vi "In Place Write String.vi"(8 "error in (no error)":errorcluster, 9 "offset (0)":i64, 10 "string in":string, 11 "pointer in":u64) -> (0 "error out":errorcluster, 1 "offset out":i64, 2 "string out":string, 3 "pointer out":u64)   [LabVIEW 2013, in "Linux RT IPC.Shared Memory.lvlib"]
uses:
  Linux RT IPC.Shared Memory.lvlib
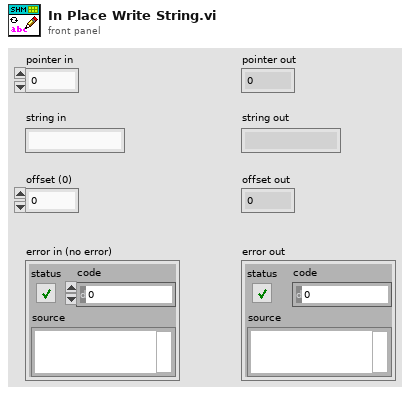
[diagram p1: front panel]
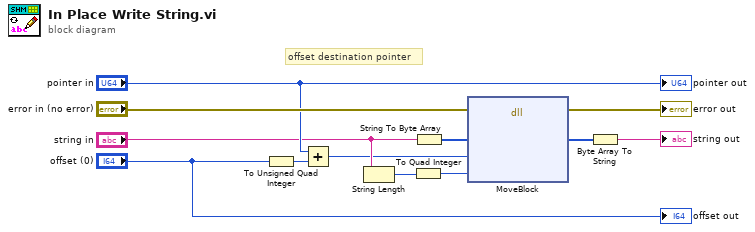
[diagram p0: block diagram]
diagram:
  # "offset destination pointer"
  n1 = To Unsigned Quad Integer(1:"offset (0)") -> (0:w6:u64)
  n2 = Add(x="pointer in", y=w6) -> (x+y=w5:u64)
  n3 = String Length(string="string in") -> (length=w3:i32)
  n4 = To Quad Integer(1:w3) -> (0:w9:i64)
  n5 = String To Byte Array(string="string in") -> (unsigned byte array=w4:u8[])
  n6 = dll-call lib="LabVIEW" fn="MoveBlock"(error in="error in (no error)", "data"=w4, "pointer"=w5, "size"=w9) -> (error out=→"error out":errorcluster, "data"=w2:u8[])  [unwired: 5 in, 1 out]
  n7 = Byte Array To String(unsigned byte array=w2) -> (string=→"string out":string)
  "pointer out" <- "pointer in"
  "offset out" <- "offset (0)"
